vi "Read Binarization treshold.vi"(8 "error in (no error)":errorcluster, 11 "Analysis params in":refnum<class "CV-Analysis.lvclass">) -> (0 "error out":errorcluster, 2 "Binarization treshold":sgl=120.0 min=0 max=255 step=1, 3 "Analysis params out":refnum<class "CV-Analysis.lvclass">)   [LabVIEW 2013, in "CameraVision.lvlib" / "CV-Analysis.lvclass"]
uses:
  CV-Analysis.lvclass
  CV-Analysis.lvclass/CV-Analysis.ctl
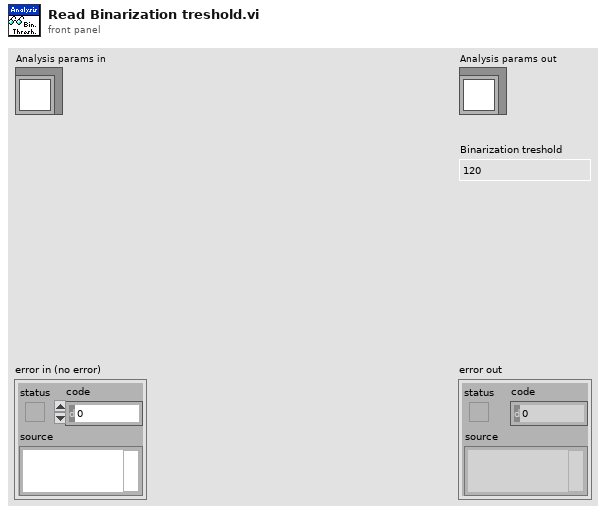
[diagram p1: front panel]
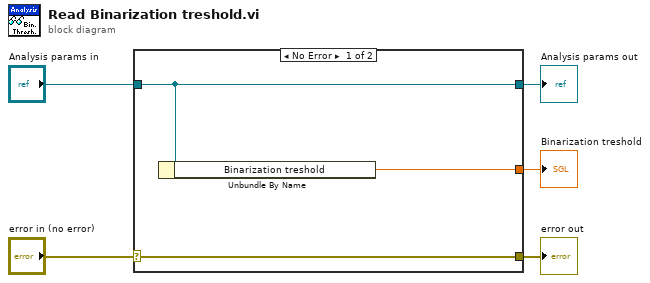
[diagram p0: block diagram]
diagram:
  n1 = case shown="No Error" "error in (no error)" {
    selector: "error in (no error)" -> [w8 w9]
    tunnel: [w8 w9] -> w4
    tunnel: [w7 w10] -> w2
    tunnel: "Analysis params in" -> [w7 w10]
    tunnel: [w6 _] -> w1
    frame No Error {
      n2 = Unbundle By Name(w7) -> ("Binarization treshold"=w6:sgl)
    }
    frame Error {
    }
  }
  "error out" <- w4
  "Analysis params out" <- w2
  "Binarization treshold" <- w1
